vi "Control - Generic - VGT Host.vi"() -> ()   [LabVIEW 2015, in "ECS-Host.lvlib"]
uses:
  ECS-Host.lvlib
  <vilib>/addons/Software Calibration Management/XControls/TBL2D.xctl
  <vilib>/addons/Software Calibration Management/XControls/TBL1D.xctl
panel:
  out "VGTPsn_PIDOut":sgl caption="[V]"
  out "MAP_Des":sgl caption="[kPa]"
  out "MAP":sgl caption="[kPa]"
  out "VGTPsn_Calc":sgl caption="[V]"
  out "ExhaustPLimited":bool caption="WGEnable"
  out "TurboSpeedLimited":bool caption="WGEnable"
  in  "ExhaustManifoldPLimit_E":bool caption="WGEnable"
  in  "TurboSpeedLimit_E":bool caption="WGEnable"
  out "VGTPsn_Des":sgl caption="[V]"
  in  "ExhaustManifoldPLimit_Tbl":cluster{"X":sgl[], "Y":sgl[]}(xcontrol)
  in  "TurboSpeedLimit_Tbl":cluster{"X":sgl[], "Y":sgl[]}(xcontrol)
  out "VGTPsn_FFTblOut":sgl caption="[V]"
  in  "VGTPsn_FFTbl":cluster{"X":sgl[], "Y":sgl[], "Z":sgl[][]}(xcontrol) caption="[]"
  in  "VGTPsn_PIDE":bool
  in  "VGTPsn_Min":sgl caption="[V]"
  in  "VGTPsn_Max":sgl caption="[V]"
  in  "VGTPsn_Man":sgl caption="[%]"
  in  "VGTPsn_ManE":bool caption="ManualBoost1SetpointEnable"
  in  "VGTPsn_Td":sgl caption="[V]"
  in  "VGTPsn_Ti":sgl caption="[V]"
  in  "VGTPsn_Kp":sgl caption="[V]"
  in  "VGTPsn_PIDMin":sgl caption="[V]"
  in  "VGTPsn_PIDMax":sgl caption="[V]"
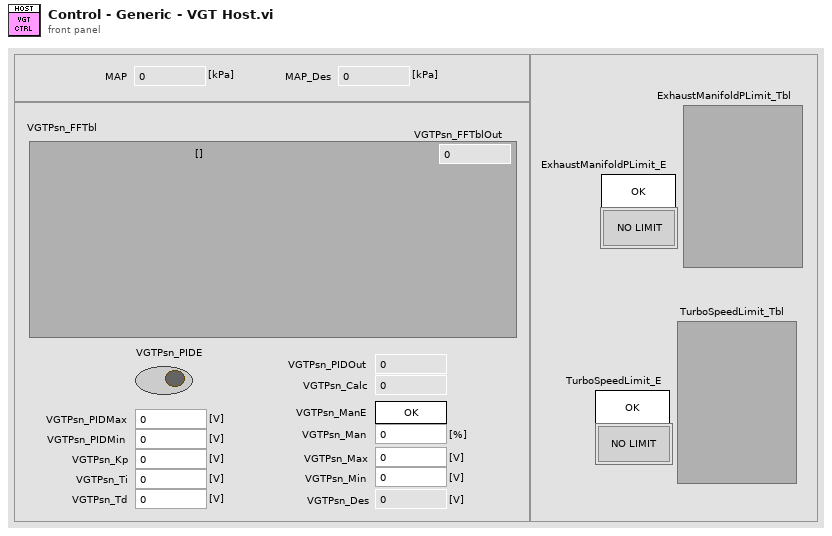
[diagram p1: front panel]
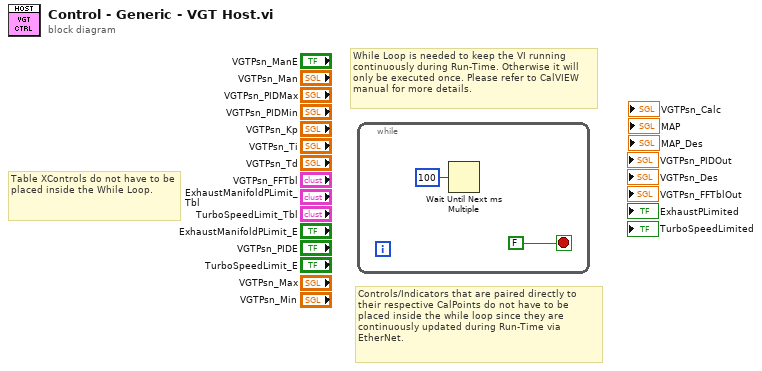
[diagram p0: block diagram]
diagram:
  # "Table XControls do not have to be placed inside the While Loop."
  # "While Loop is needed to keep the VI running\ncontinuously during Run-Time. Otherwise it will only be executed once. Please refer to CalVIEW manual for more details."
  # "Controls/Indicators that are paired directly to their respective CalPoints do not have to be placed inside the while loop since they are continuously updated during Run-Time via EtherNet."
  n1 = while {
    stop <- FALSE stop-if-true
    n2 = Wait Until Next ms Multiple(millisecond multiple=u32 100) -> ()  [unwired: 1 out]
  }
